vi "CRYReport Model LIB.vi"(7 "sAction":string, 8 "nData":i32, 9 "sData":string) -> (0 "nData_Out":i32, 1 "sData_Out":string)   [LabVIEW 2013]
uses:
  CRYReport Global.vi
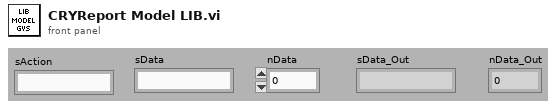
[diagram p1: front panel]
types:
  T1 = cluster{"nID":i16, "sName":string, "pVIRef":refnum<vi>, "pSPRef":refnum<vi>, "sTitle":string, "nIDObject":i16, "nIDV":i16, "nWidth":i16, "nHeight":i16, "bImgChange":bool, "sType":string, "sState":string, "sPosition":string, "sData":string}
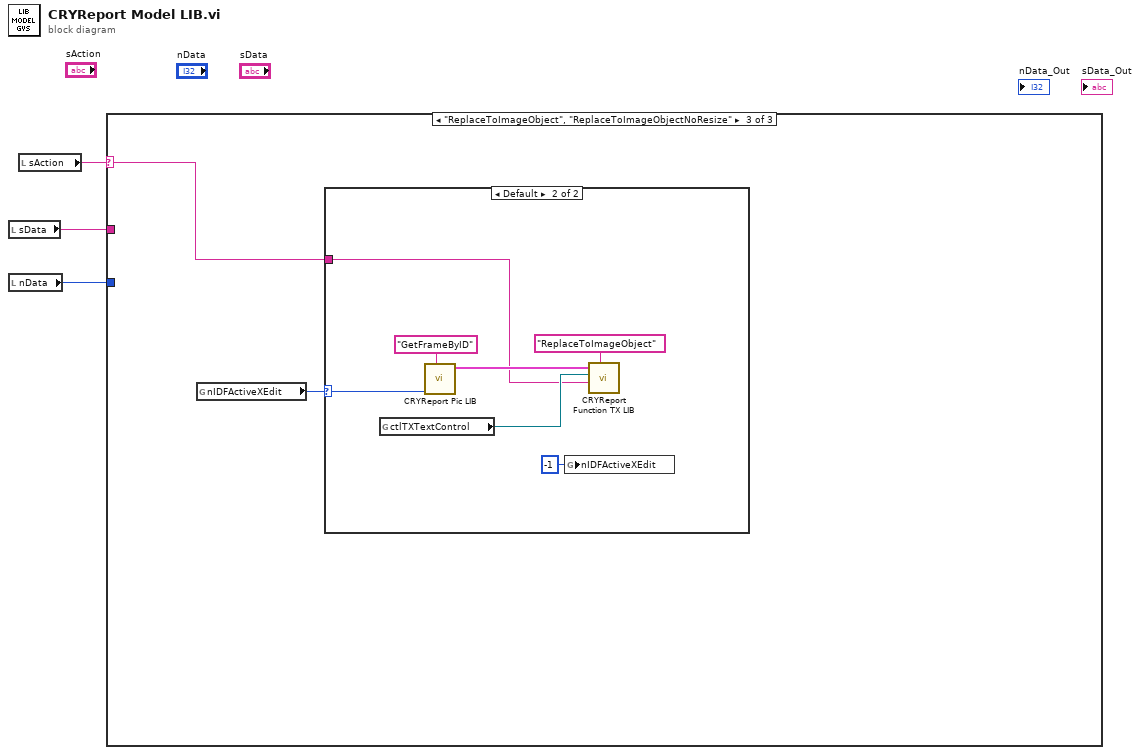
[diagram p0: block diagram]
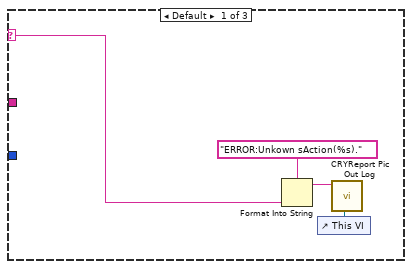
[diagram p2: hidden frame]
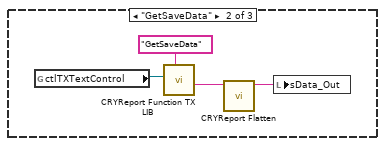
[diagram p3: hidden frame]
diagram:
  n1 = local read "sData"() -> (w2:string)
  n2 = local read "nData"() -> (w1:i32)
  n3 = local read "sAction"() -> (w3:string)
  n4 = case shown="\"ReplaceToImageObject\", \"ReplaceToImageObjectNoResize\"" w3 {
    selector: w3 -> [w5 _ w12]
    tunnel: w2 -> [_ _ _]
    tunnel: w1 -> [_ _ _]
    frame Default {
      n5 = Format Into String(format string="ERROR:Unkown sAction(%s).", w5) -> (resulting string=w4:string)  [unwired: 2 in, 1 out]
      n6 = control-ref of="This VI"() -> (w7:refnum<vi>)
      n7 = call "CRYReport Pic Out Log.vi"("vi reference"=w7, "sData"=w4) -> ()  [unwired: 10 in]
    }
    frame "GetSaveData" {
      n8 = global read "CRYReport Global.vi" "ctlTXTextControl"() -> (w10:refnum<k7>)
      n9 = call "CRYReport Function TX LIB.vi"("sAction"="GetSaveData", "TXTextControl"=w10) -> ("sData_Out"=w9:string)  [unwired: 7 in, 2 out]
      n10 = call "CRYReport Flatten.vi"("sData"=w9) -> ("flattened Data"=w8:string)  [unwired: 10 in]
      n11 = local write "sData_Out"(w8) -> ()
    }
    frame "ReplaceToImageObject", "ReplaceToImageObjectNoResize" {
      n12 = global read "CRYReport Global.vi" "nIDFActiveXEdit"() -> (w13:i16)
      n13 = case shown="Default" w13 {
        selector: w13 -> [_ w18]
        tunnel: w12 -> [_ w14]
        frame -1 {
        }
        frame Default {
          n14 = global read "CRYReport Global.vi" "ctlTXTextControl"() -> (w15:refnum<k7>)
          n15 = call "CRYReport Pic LIB.vi"("sAction"="GetFrameByID", "nData"=w18) -> ("cFrame_Out"=w16:T1)  [unwired: 6 in, 3 out]
          n16 = global write "CRYReport Global.vi" "nIDFActiveXEdit"(i16 -1 ("nIDFActiveXEdit")) -> ()
          n17 = call "CRYReport Function TX LIB.vi"("sAction"="ReplaceToImageObject", "sData"=w14, "TXTextControl"=w15, "cFrame"=w16) -> ()  [unwired: 5 in, 3 out]
        }
      }
    }
  }
